vi "Set Data Test.vi"(8 "error in (no error)":errorcluster caption="entrée d'erreur (pas d'erreur)", 10 "Data_Test Read":T1(array[cluster]), 11 "Database Altyor en entrée":refnum<class "Database Altyor.lvclass">) -> (0 "error out":errorcluster caption="sortie d'erreur", 3 "Database Altyor en sortie":refnum<class "Database Altyor.lvclass">)   [LabVIEW 2020, in "Library Instrument & Equipement.lvlib" / "Library Database.lvlib" / "Database Altyor.lvclass"]
uses:
  Database Altyor.lvclass
  Database Altyor.lvclass/Database Altyor.ctl
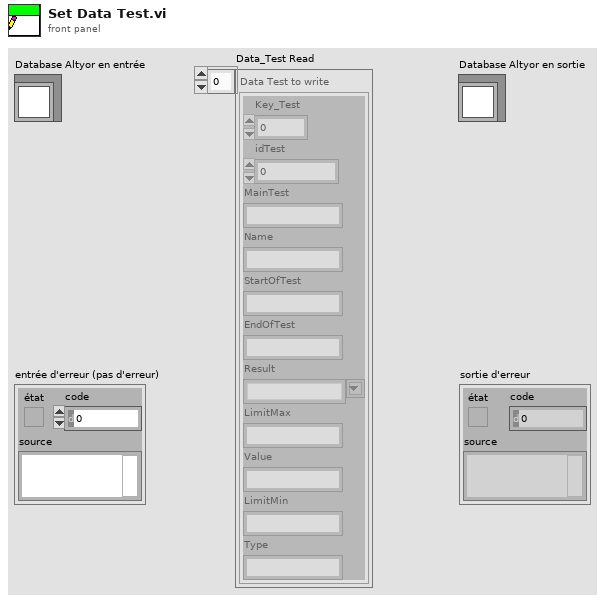
[diagram p1: front panel]
types:
  T1 = cluster{"Key_Test":u32, "idTest":u32, "MainTest":string, "Name":string, "StartOfTest":string, "EndOfTest":string, "Result":string, "LimitMax":string, "Value":string, "LimitMin":string, "Type":string}[]
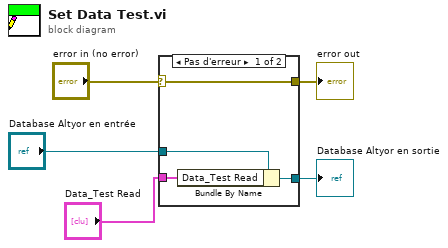
[diagram p0: block diagram]
diagram:
  n1 = case shown="Pas d'erreur" "error in (no error)" {
    selector: "error in (no error)" -> [w9 w10]
    tunnel: [w9 w10] -> w4
    tunnel: [w7 w11] -> w2
    tunnel: "Database Altyor en entrée" -> [w8 w11]
    tunnel: "Data_Test Read" -> [w6 _]
    frame No Error {
      n2 = Bundle By Name(cluster=w8, "Data_Test Read"=w6) -> (w7:refnum<class "Database Altyor.lvclass">)
    }
    frame Error {
    }
  }
  "error out" <- w4
  "Database Altyor en sortie" <- w2
